vi "Send Write Sine Wave.vi"(7 "Priority":T2=enum."Normal" caption="Message Priority (Normal)", 8 "error in (no error)":errorcluster, 10 "Sin Wave Parameters":T1={"phase"=0.0, "amplitude"=1.0, "frequency"=10.0, "offset"=0.0} {"offset" format="%#_13g"; "frequency" format="%0.2p"; "amplitude" format="%0.2p"; "phase" format="%.2p"}, 11 "Message Enqueuer in":refnum<class "Message Enqueuer.lvclass">) -> (0 "error out":errorcluster, 3 "Message Enqueuer out":refnum<class "Message Enqueuer.lvclass">)   [LabVIEW 2015, in "Analog Output Channel.lvlib" / "Write Sine Wave Msg.lvclass"]
doc: "Sends the <b>Analog Output Channel.lvlib:Write Sine Wave Msg.lvclass</b> message.\n\nThis message will call <b>Write Sine Wave.vi</b> on the <b>Analog Output Channel.lvlib:Analog Output Channel.lvclass</b> actor.\n\n<b>Write Sine Wave.vi Description</b>"
uses:
  Write Sine Wave Msg.lvclass
  <vilib>/ActorFramework/Message Enqueuer/Message Enqueuer.lvclass
  <vilib>/ActorFramework/Message Enqueuer/Message Priority.ctl
  Write Sine Wave Msg.lvclass/Write Sine Wave Msg.ctl
  <vilib>/ActorFramework/Message Enqueuer/Message Enqueuer.lvclass/Message Enqueuer.ctl
  <vilib>/ActorFramework/Message Priority Queue/Priority Enqueue.vi
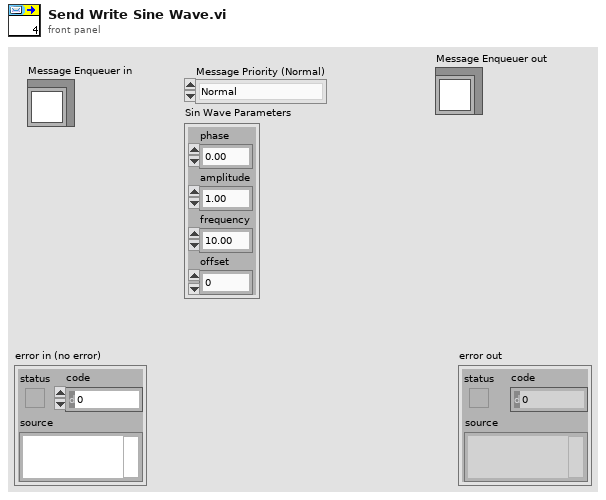
[diagram p1: front panel]
types:
  T1 = cluster{"phase":dbl, "amplitude":dbl, "frequency":dbl, "offset":dbl}
  T2 = typedef "Actor Framework.lvlib/Message Enqueuer.lvclass/Message Priority.ctl" = enum16{"Low", "Normal", "High"}
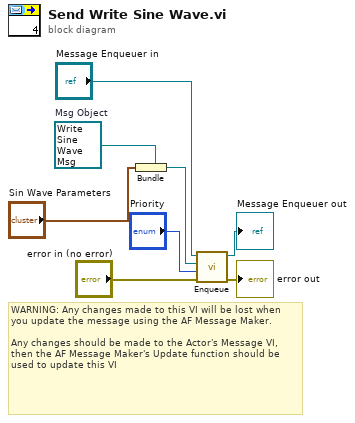
[diagram p0: block diagram]
diagram:
  w7 = refnum<class "Write Sine Wave Msg.lvclass"> refnum  # Msg Object
  # "WARNING: Any changes made to this VI will be lost when you update the message using the AF Message Maker.\n\nAny changes should be made to the Actor's Message VI, then the AF Message Maker's Update function should be used to update this VI"
  n1 = Bundle(cluster=w7, "Sin Wave Parameters") -> (w2:refnum<class "Write Sine Wave Msg.lvclass">)
  n2 = call <vilib>:"Enqueue.vi"("error in (no error)"="error in (no error)", "Message Priority (Normal)"="Priority", "Message"=w2, "Message Enqueuer in"="Message Enqueuer in") -> ("error out"=→"error out":errorcluster, "Message Enqueuer out"=→"Message Enqueuer out":refnum<class "Message Enqueuer.lvclass">)  [unwired: 6 in]
